vi "CreateIlluminationMask.vi"(8 "error in (no error)":errorcluster, 9 "Image trig":u16[](array[numeric]), 10 "Time at P_f":u32[](array[numeric]), 11 "Final step, n":u16[](array[numeric])) -> (0 "error out":errorcluster, 1 "Image trig OUT":u16[](array[numeric]), 2 "Time at P_f OUT":u32[](array[numeric]), 3 "Final step OUT":u16[](array[numeric]))   [LabVIEW 2016]
uses:
  <vilib>/Utility/Variable/NI_VariableUtilities.lvlib
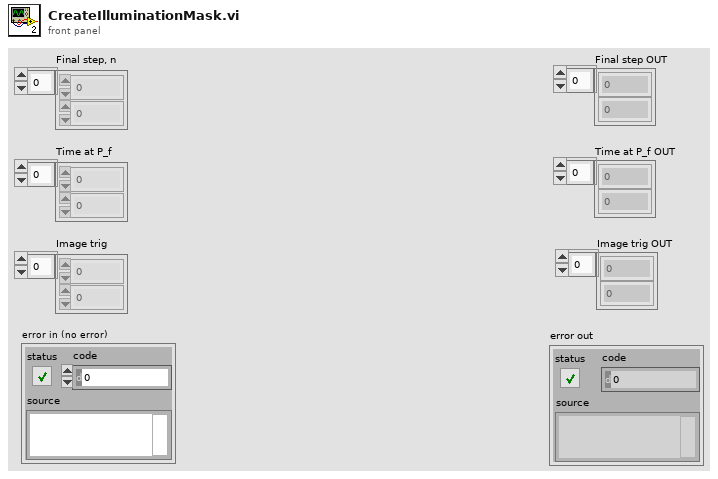
[diagram p1: front panel]
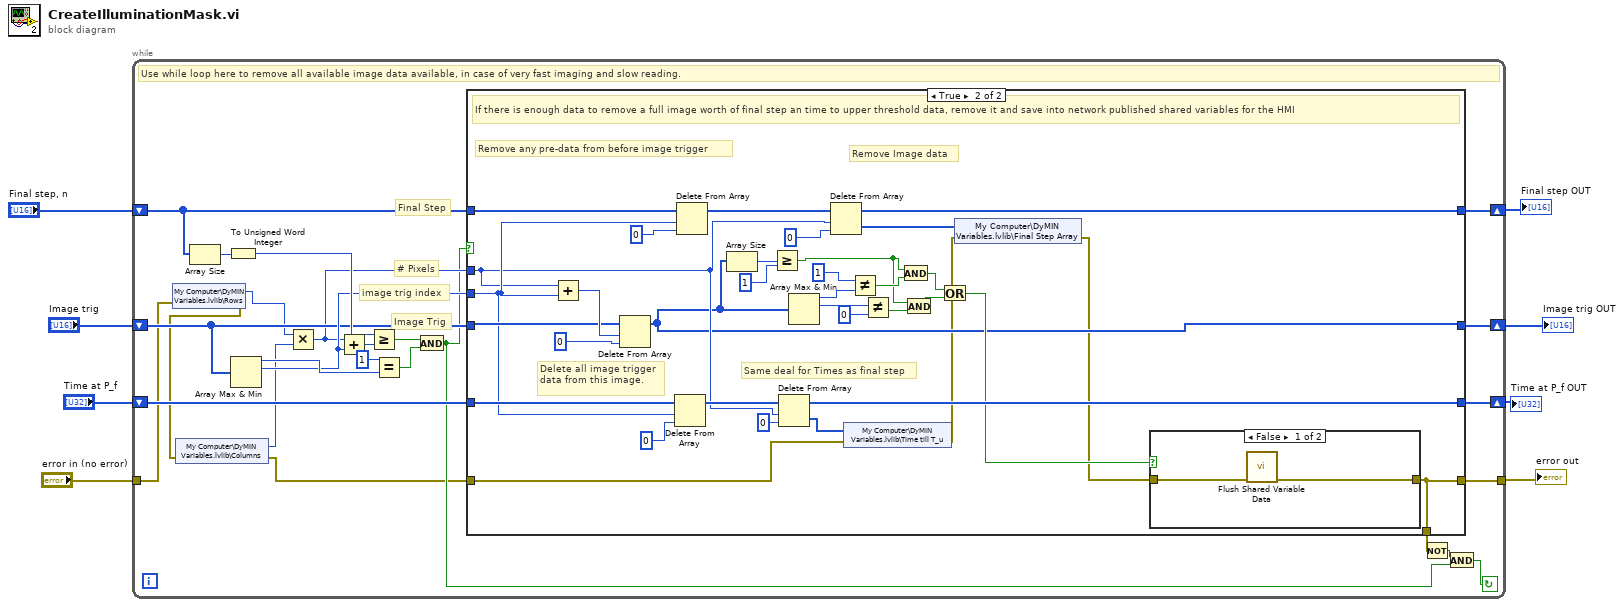
[diagram p0: block diagram]
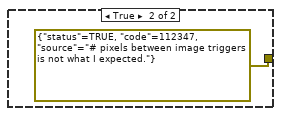
[diagram p3: hidden frame]
diagram:
  n1 = while {
    shift-right: [w25] -> w7
    shift-left: "Final step, n" -> [w26]
    shift-right: [w22] -> w5
    shift-left: "Image trig" -> [w23]
    shift-right: [w20] -> w4
    shift-left: "Time at P_f" -> [w19]
    tunnel: "error in (no error)" -> [w11]
    tunnel: [w18] -> w1
    stop <- w14 continue-if-true
    # "# Pixels"
    # "Image Trig"
    # "image trig index"
    # "Final Step"
    # "Use while loop here to remove all available image data available, in case of very fast imaging and slow reading."
    n2 = shared-variable "My Computer\\DyMIN Variables.lvlib\\Rows"(error in=w11) -> (w13:i32, error out=w10:errorcluster)
    n3 = shared-variable "My Computer\\DyMIN Variables.lvlib\\Columns"(error in=w10) -> (w12:i32, error out=w9:errorcluster)
    n4 = Array Size(array=w26) -> (size(s)=w33:i32)
    n5 = To Unsigned Word Integer(number=w33) -> (unsigned 16bit integer=w32:u16)
    n6 = Array Max & Min(array=w23) -> (max value=w30:u16, max index (indices)=w24:i32)  [unwired: 2 out]
    n7 = Multiply(x=w13, y=w12) -> (x*y=w21:i32)
    n8 = Add(x=w21, y=w24) -> (x+y=w29:i32)
    n9 = Greater Or Equal?(x=w32, y=w29) -> (x >= y?=w28:bool)
    n10 = Equal?(x=u16 1, y=w30) -> (x = y?=w27:bool)
    n11 = And(x=w28, y=w27) -> (x .and. y?=w15:bool)
    n12 = case shown="True" w15 {
      tunnel: w26 -> [w37 w71]
      tunnel: w9 -> [w34 w40]
      tunnel: w19 -> [w35 w70]
      tunnel: [w34 w44] -> w18
      tunnel: [w37 w51] -> w25
      tunnel: w23 -> [w36 w66]
      tunnel: [w36 w43] -> w22
      tunnel: [w35 w59] -> w20
      tunnel: w24 -> [_ w63]
      tunnel: w21 -> [_ w60]
      tunnel: [w34 w44] -> w17
      frame False {
        # "If there isn't enough data to build a full image yet, just pass it through."
      }
      frame True {
        # "Delete all image trigger data from this image."
        # "Same deal for Times as final step"
        # "Remove Image data"
        # "Remove any pre-data from before image trigger"
        # "If there is enough data to remove a full image worth of final step an time to upper threshold data, remove it and save into network published shared variables for the HMI"
        n13 = Add(x=w60, y=w63) -> (x+y=w67:i32)
        n14 = Delete From Array(array=w66, length=w67, index=0) -> (array with subset deleted=w43:u16[])  [unwired: 1 out]
        n15 = Delete From Array(array=w70, length=w63, index=0) -> (array with subset deleted=w62:u32[])  [unwired: 1 out]
        n16 = Delete From Array(array=w71, length=w63, index=0 ("length")) -> (array with subset deleted=w54:u16[])  [unwired: 1 out]
        n17 = Array Size(array=w43) -> (size(s)=w53:i32)
        n18 = Greater Or Equal?(x=w53, y=1) -> (x >= y?=w48:bool)
        n19 = Delete From Array(array=w62, length=w60, index=0) -> (deleted portion=w41:u32[], array with subset deleted=w59:u32[])
        n20 = Array Max & Min(array=w43) -> (max value=w58:u16, max index (indices)=w55:i32)  [unwired: 2 out]
        n21 = Delete From Array(array=w54, length=w60, index=0) -> (deleted portion=w42:u16[], array with subset deleted=w51:u16[])
        n22 = shared-variable "My Computer\\DyMIN Variables.lvlib\\Time till T_u"(w41, error in=w40) -> (error out=w39:errorcluster)
        n23 = Not Equal?(x=u16 1, y=w58) -> (x != y?=w50:bool)
        n24 = Not Equal?(x=w55, y=0 ("max index(es)")) -> (x != y?=w47:bool)
        n25 = And(x=w48, y=w50) -> (x .and. y?=w46:bool)
        n26 = And(x=w48, y=w47) -> (x .and. y?=w49:bool)
        n27 = Or(x=w46, y=w49) -> (x .or. y?=w45:bool)
        n28 = shared-variable "My Computer\\DyMIN Variables.lvlib\\Final Step Array"(w42, error in=w39) -> (error out=w38:errorcluster)
        n29 = case shown="False" w45 {
          tunnel: [w72 errorcluster {"status"=TRUE, "code"=112347, "source"="# pixels between image triggers is not what I expected."} ("error constant")] -> w44
          tunnel: w38 -> [w73 _]
          frame False {
            n30 = call <vilib>:"Flush Shared Variable Data.vi"("error in (no error)"=w73) -> ("error out"=w72:errorcluster)  [unwired: 10 in]
          }
          frame True {
          }
        }
      }
    }
    n31 = Not(x=w17) -> (.not. x?=w16:bool)
    n32 = And(x=w16, y=w15) -> (x .and. y?=w14:bool)
  }
  "Final step OUT" <- w7
  "Image trig OUT" <- w5
  "Time at P_f OUT" <- w4
  "error out" <- w1
